vi "Project Tree Drag Over.vi"(8 "error in (no error)":errorcluster, 9 "Available Data Names":string[](array[string]), 10 "Coords":T1, 11 "TreeControl in":refnum<vi>) -> (0 "error out":errorcluster, 1 "Accepted":bool, 3 "TreeControl out":refnum<vi>)   [LabVIEW 2015, in "Editor.lvclass"]
uses:
  Editor.lvclass
  <vilib>/Utility/miscctls.llb/LVPoint32TypeDef.ctl
panel:
  out "Tag":string
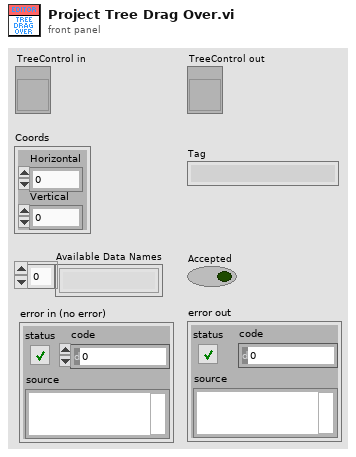
[diagram p1: front panel]
types:
  T1 = typedef "LVPoint32TypeDef.ctl" = cluster{"Horizontal":i32, "Vertical":i32}
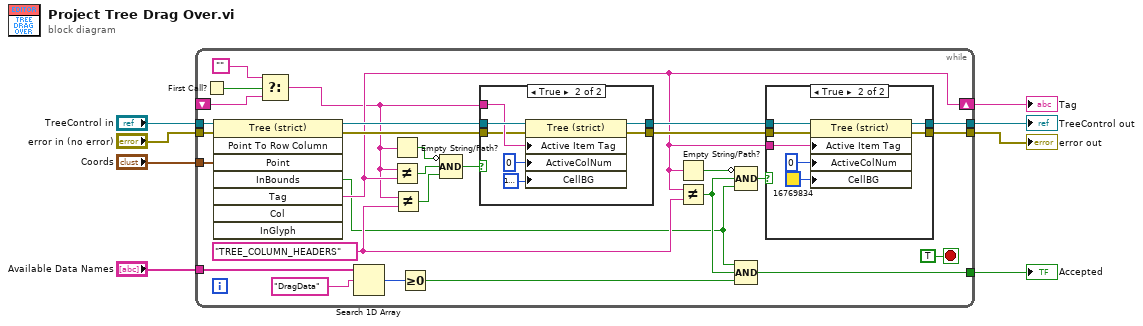
[diagram p0: block diagram]
diagram:
  n1 = while {
    tunnel: "Coords" -> [w30]
    tunnel: "TreeControl in" -> [w29]
    tunnel: [w9] -> w1
    tunnel: "Available Data Names" -> [w26]
    tunnel: "error in (no error)" -> [w25]
    shift-right: [w14] -> w4
    shift-left: _ -> [w15]
    tunnel: [w23] -> w3
    tunnel: [w22] -> w2
    stop <- TRUE stop-if-true
    w13 = "TREE_COLUMN_HEADERS"
    n2 = First Call?() -> (First Call?: T/F=w17:bool)
    n3 = invoke class="Tree (strict)" method="Point To Row Column"(reference=w29, error in=w25, "Point"=w30) -> (reference out=w34:refnum<vi>, error out=w35:errorcluster, "InBounds"=w11:bool, "Tag"=w14:string)  [unwired: 5 in, 4 out]
    n4 = Select(t="", s=w17, f=w15) -> (s? t:f=w10:string)
    n5 = Search 1D Array(1D array=w26, element="DragData" ("data name")) -> (index of element=w28:i32)  [unwired: 1 in]
    n6 = Empty String/Path?(string/path=w10) -> (empty?=w32:bool)
    n7 = Not Equal?(x=w10, y=w14) -> (x != y?=w31:bool)
    n8 = Not Equal?(x=w10, y=w13) -> (x != y?=w12:bool)
    n9 = Greater Or Equal To 0?(x=w28) -> (x >= 0?=w18:bool)
    n10 = Compound Arithmetic op=AND(invert w32, w31, w12) -> (w33:bool)
    n11 = case shown="True" w33 {
      tunnel: w34 -> [w39 w46]
      tunnel: w10 -> [_ w45]
      tunnel: w35 -> [w38 w44]
      tunnel: [w39 w41] -> w37
      tunnel: [w38 w40] -> w36
      frame False {
      }
      frame True {
        n12 = property class="Tree (strict)"(reference=w46, error in=w44, "Active Item Tag"=w45, "ActiveColNum"=0 ("Active Cell:Active Column Number"), "CellBG"=u32 16777216) -> (reference out=w41:refnum<vi>, error out=w40:errorcluster)
      }
    }
    n13 = Empty String/Path?(string/path=w14) -> (empty?=w21:bool)
    n14 = Not Equal?(x=w14, y=w13) -> (x != y?=w19:bool)
    n15 = Compound Arithmetic op=AND(invert w21, w19, w11) -> (w20:bool)
    n16 = Compound Arithmetic op=AND(w11, w19, w18) -> (w9:bool)
    n17 = case shown="True" w20 {
      tunnel: w37 -> [w48 w55]
      tunnel: w36 -> [w47 w54]
      tunnel: w14 -> [_ w53]
      tunnel: [w48 w50] -> w23
      tunnel: [w47 w49] -> w22
      frame False {
      }
      frame True {
        n18 = property class="Tree (strict)"(reference=w55, error in=w54, "Active Item Tag"=w53, "ActiveColNum"=0 ("Active Cell:Active Column Number"), "CellBG"=u32 16769834) -> (reference out=w50:refnum<vi>, error out=w49:errorcluster)
      }
    }
  }
  "Accepted" <- w1
  "TreeControl out" <- w3
  "error out" <- w2
  "Tag" <- w4
